vi "Control Ref Filter.vi"(1 "Controls[]":refnum<vi>[](array[refnum])) -> (0 "valide controls":refnum<vi>[](array[refnum]))   [LabVIEW 2016]
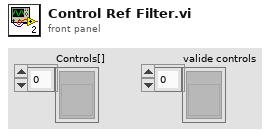
[diagram p1: front panel]
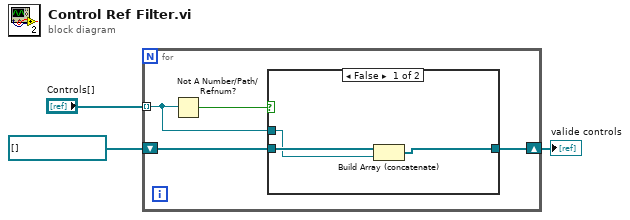
[diagram p0: block diagram]
diagram:
  n1 = for {
    shift-right: [w6] -> w3
    shift-left: refnum<vi>[] [] ("Controls[]") -> [w5]
    tunnel: "Controls[]" -> [w4] mode=indexing
    n2 = Not A Number/Path/Refnum?(number/path/refnum=w4) -> (NaN/Path/Refnum?=w7:bool)
    n3 = case shown="False" w7 {
      tunnel: [w8 w11] -> w6
      tunnel: w5 -> [w10 w11]
      tunnel: w4 -> [w9 _]
      frame False {
        n4 = Build Array (concatenate)(w10, w9) -> (w8:refnum<vi>[])
      }
      frame True {
      }
    }
  }
  "valide controls" <- w3
